vi "Example Circular Buffer (Producer-Monitor).vi"() -> ()   [LabVIEW 2013]
uses:
  VariantBuffer/VariantBuffer.lvclass
panel:
  out "data":string[](array[string])
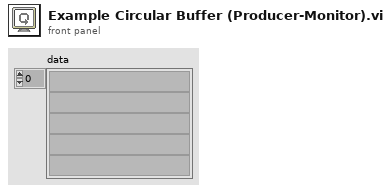
[diagram p1: front panel]
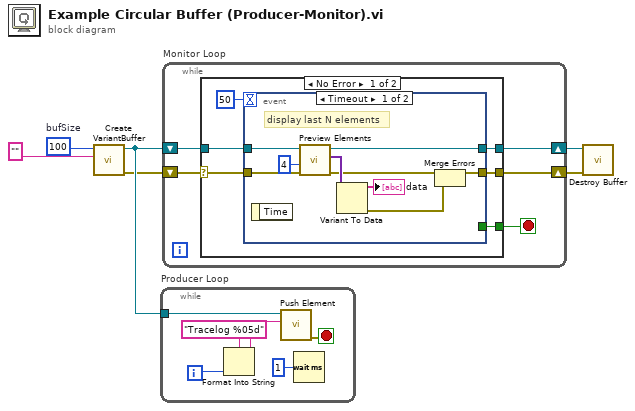
[diagram p0: block diagram]
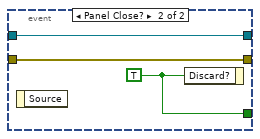
[diagram p2: hidden frame]
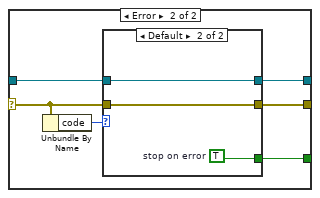
[diagram p3: hidden frame]
diagram:
  w6 = 100  # bufSize
  n1 = call "Create VariantBuffer.vi"("default"="", "bufSize"=w6) -> ("error out"=w2:errorcluster, "Buffer"=w4:refnum<data-value>)  [unwired: 8 in]
  n2 = while "Producer Loop" {
    tunnel: w4 -> [w9]
    i -> [w11]
    stop <- w7 stop-if-true
    n3 = Format Into String(format string="Tracelog %05d", w11) -> (resulting string=w8:string)  [unwired: 2 in, 1 out]
    n4 = call "Push Element.vi"("element"=w8, "Buffer in"=w9) -> ("error out"=w7:errorcluster)  [unwired: 8 in, 1 out]
    n5 = Wait (ms)(milliseconds to wait=u32 1) -> ()  [unwired: 1 out]
  }
  n6 = while "Monitor Loop" {
    shift-right: [w16] -> w3
    shift-left: w4 -> [w17]
    shift-right: [w15] -> w1
    shift-left: w2 -> [w13]
    stop <- w14 stop-if-true
    n7 = case shown="No Error" w13 {
      selector: w13 -> [w18 w37]
      tunnel: w17 -> [w22 w38]
      tunnel: [w21 w39] -> w16
      tunnel: [w20 w36] -> w15
      tunnel: [w19 w41] -> w14
      frame No Error {
        n8 = event shown="[0] Timeout" {
          selector: _ -> [_ _]
          dyn-events: _ -> [_ _]
          timeout: 50 -> [_ _]
          tunnel: w22 -> [w31 w35]
          tunnel: [w30 w35] -> w21
          tunnel: [_ w34] -> w19
          tunnel: w18 -> [w27 w33]
          tunnel: [w26 w33] -> w20
          event Timeout {
            # "display last N elements"
            n9 = event-data() -> ()  [unwired: 1 in, 1 out]
            n10 = call "Preview Elements.vi"("error in"=w27, "count (-1: all)"=4, "ByteBuffer in"=w31) -> ("error out"=w25:errorcluster, "elements"=w28:variant[], "ByteBuffer"=w30:refnum<data-value>)  [unwired: 6 in]
            n11 = Variant To Data(Variant=w28) -> (data=→"data":string[], error out=w24:errorcluster)  [unwired: 2 in]
            n12 = Merge Errors(w25, w24) -> (w26:errorcluster)
          }
          event Panel Close? {
            w34 = TRUE ("Discard?")
            n13 = event-data() -> ()  [unwired: 1 in, 1 out]
            n14 = event-data("Discard?"=w34) -> ()  [unwired: 1 in, 1 out]
          }
        }
      }
      frame Error {
        n15 = Unbundle By Name(w37) -> ("code"=w40:i32)
        n16 = case shown="Default" w40 {
          tunnel: [_ w45] -> w41
          tunnel: [w42 w44] -> w39
          tunnel: w38 -> [w42 w44]
          tunnel: w37 -> [_ w43]
          tunnel: [_ w43] -> w36
          frame 0 {
            # "Handle Error\n& Continue"
          }
          frame Default {
            w45 = TRUE  # stop on error
          }
        }
      }
    }
  }
  n17 = call "Destroy Buffer.vi"("error in"=w1, "Buffer"=w3) -> ()  [unwired: 8 in, 2 out]
